vi "Scripting.vi"() -> ()   [LabVIEW 2019]
uses:
  NationalInstruments.VeriStand.SystemDefinitionAPI
  <vilib>/NI VeriStand/Custom Device API/Custom Device Item Ref.ctl
  Addon/Support Libraries/Protocols.lvlibp/Protocol Parent/Protocol Parent.lvclass
  Addon/Support Libraries/Protocols.lvlibp/TCP/TCP.lvclass
  Addon/Support Libraries/Protocols.lvlibp/UDP/UDP.lvclass
  Scripting API/Polymorphic/Create Message_TriggerOnly.vi
  Scripting API/Polymorphic/Create Message_PeriodicAndTrigger.vi
  Scripting API/Polymorphic/Create Message_ValueChangeAndTrigger.vi
  Scripting API/Polymorphic/Create Channel/Create Global Command Single Channel_Format.vi
  Scripting API/Polymorphic/Create Channel/Create Command Array Channel_Type Cast.vi
  Scripting API/Polymorphic/Add Response_Byte count.vi
  Scripting API/Polymorphic/Add Response_Wait sec.vi
  Scripting API/Polymorphic/Create Channel/Create Response Single Channel_Comparison.vi
  Scripting API/Scripting API.lvlib
  <vilib>/NI VeriStand/Custom Device API/Custom Device API.lvlib
  Scripting API/Polymorphic/Create RS-xxx.vi
  Scripting API/Polymorphic/Create TCP.vi
panel:
  out "Message refnum out 6":T1=18446744073709551615 format="%.0x"
  out "Channel refnum out 2":T1=18446744073709551615 format="%.0x"
  out "error out 17":errorcluster
  in  "Message refnum in 3":T1=18446744073709551615 format="%.0x"
  in  "Expected String":string
  in  "error in (no error) 17":errorcluster
  in  "Default Value 2":dbl
  in  "Units 2":string
  out "UDP out":refnum<class "UDP.lvclass">
  out "error out 13":errorcluster
  in  "error in (no error) 13":errorcluster
  out "TCP out":refnum<class "TCP.lvclass">
  out "error out 10":errorcluster
  in  "error in (no error) 10":errorcluster
  out "Response refnum out 2":T1=18446744073709551615 format="%.0x"
  out "error out 9":errorcluster
  in  "Response refnum in 2":T1=18446744073709551615 format="%.0x"
  in  "Response 2":string
  in  "Linkages 2":T2(array[cluster]) {"Linked Channel refnum" format="%.0x"}
  in  "error in (no error) 9":errorcluster
  in  "Wait value":dbl
  in  "Channel refnum 2":T1=18446744073709551615 format="%.0x"
  out "Response refnum out":T1=18446744073709551615 format="%.0x"
  out "error out 8":errorcluster
  in  "Response refnum in":T1=18446744073709551615 format="%.0x"
  in  "Response":string
  in  "Linkages":T2(array[cluster]) {"Linked Channel refnum" format="%.0x"}
  in  "error in (no error) 8":errorcluster
  in  "Byte Count value":u32
  in  "Channel refnum":T1=18446744073709551615 format="%.0x"
  out "Target out 4":refnum<k24>
  out "Instrument Addon Custom Device refnum 4":T1=18446744073709551615 format="%.0x"
  out "Message Channels refnums 4":T3 {"Enable Periodic" format="%.0x"; "Error Code" format="%.0x"; "Message Status" format="%.0x"; "Timestamp" format="%.0x"; "Trigger" format="%.0x"}
  out "error out 16":errorcluster
  in  "Target in 4":refnum<k24>
  in  "Protocol in":refnum<class "Protocol Parent.lvclass">
  in  "PCL Decimation 3":u16
  in  "error in (no error) 16":errorcluster
  out "Channel refnums out":T1[](array[typedef]) format="%.0x"
  out "Channel refnum out":T1=18446744073709551615 format="%.0x"
  out "Message refnum out 5":T1=18446744073709551615 format="%.0x"
  out "error out 15":errorcluster
  in  "Message refnum in 2":T1=18446744073709551615 format="%.0x"
  in  "Type":enum16{"DBL"}(ring)
  in  "Endian":enum16{"Big", "Little", "Native"}(ring)
  in  "error in (no error) 15":errorcluster
  in  "Delimiter":string
  out "Instrument Addon refnum out 3":T1=18446744073709551615 format="%.0x"
  out "error out 14":errorcluster
  in  "Instrument Addon refnum in 3":T1=18446744073709551615 format="%.0x"
  in  "Format String":string
  in  "error in (no error) 14":errorcluster
  in  "Default Value":dbl
  in  "Units":string
  in  "Trigger Channel refnum 3":T1=18446744073709551615 format="%.0x"
  in  "Enable Periodic Default ON 3":bool
  in  "Trigger Channel refnum 2":T1=18446744073709551615 format="%.0x"
  in  "Enable Periodic Default ON 2":bool
  in  "Trigger Channel refnum":T1=18446744073709551615 format="%.0x"
  in  "Enable Periodic Default ON":bool
  out "Message Channels refnums 3":T3 {"Enable Periodic" format="%.0x"; "Error Code" format="%.0x"; "Message Status" format="%.0x"; "Timestamp" format="%.0x"; "Trigger" format="%.0x"}
  out "Message Channels refnums 2":T3 {"Enable Periodic" format="%.0x"; "Error Code" format="%.0x"; "Message Status" format="%.0x"; "Timestamp" format="%.0x"; "Trigger" format="%.0x"}
  out "Message Channels refnums":T3 {"Enable Periodic" format="%.0x"; "Error Code" format="%.0x"; "Message Status" format="%.0x"; "Timestamp" format="%.0x"; "Trigger" format="%.0x"}
  out "Message Group refnum out 4":T1=18446744073709551615 format="%.0x"
  out "Message refnum out 4":T1=18446744073709551615 format="%.0x"
  out "error out 12":errorcluster
  in  "Message Group refnum in 3":T1=18446744073709551615 format="%.0x"
  in  "Message name 3":string
  in  "Protection 3":T4(ring)
  in  "error in (no error) 12":errorcluster
  out "Message Group refnum out 3":T1=18446744073709551615 format="%.0x"
  out "Message refnum out 3":T1=18446744073709551615 format="%.0x"
  out "error out 11":errorcluster
  in  "Message Group refnum in 2":T1=18446744073709551615 format="%.0x"
  in  "Message name 2":string
  in  "Protection 2":T4(ring)
  in  "error in (no error) 11":errorcluster
  in  "Period (sec)":u32
  out "Message Group refnum out 2":T1=18446744073709551615 format="%.0x"
  out "Message refnum out":T1=18446744073709551615 format="%.0x"
  out "error out 6":errorcluster
  in  "Message Group refnum in":T1=18446744073709551615 format="%.0x"
  in  "Message name":string
  in  "error in (no error) 6":errorcluster
  out "Command refnum out":T1=18446744073709551615 format="%.0x"
  out "Message refnum out 2":T1=18446744073709551615 format="%.0x"
  out "error out 7":errorcluster
  in  "Message refnum in":T1=18446744073709551615 format="%.0x"
  in  "Command":string
  in  "error in (no error) 7":errorcluster
  out "Instrument Addon refnum out 2":T1=18446744073709551615 format="%.0x"
  out "Message Group refnum out":T1=18446744073709551615 format="%.0x"
  out "error out 5":errorcluster
  in  "Instrument Addon refnum in 2":T1=18446744073709551615 format="%.0x"
  in  "Message Group name":string
  in  "error in (no error) 5":errorcluster
  out "Instrument Addon refnum out":T1=18446744073709551615 format="%.0x"
  out "error out 4":errorcluster
  in  "Instrument Addon refnum in":T1=18446744073709551615 format="%.0x"
  in  "Exported File path":path
  in  "error in (no error) 4":errorcluster
  out "Target out 3":refnum<k24>
  out "Instrument Addon Custom Device refnum 3":T1=18446744073709551615 format="%.0x"
  out "error out 3":errorcluster
  in  "Target in 3":refnum<k24>
  in  "Config File Path":path
  in  "error in (no error) 3":errorcluster
  out "Target out 2":refnum<k24>
  out "Instrument Addon Custom Device refnum 2":T1=18446744073709551615 format="%.0x"
  out "error out 2":errorcluster
  in  "Target in 2":refnum<k24>
  in  "PCL Decimation 2":u16
  in  "error in (no error) 2":errorcluster
  out "Target out":refnum<k24>
  out "Instrument Addon Custom Device refnum":T1=18446744073709551615 format="%.0x"
  out "error out":errorcluster
  in  "Target in":refnum<k24>
  in  "PCL Decimation":u16
  in  "error in (no error)":errorcluster
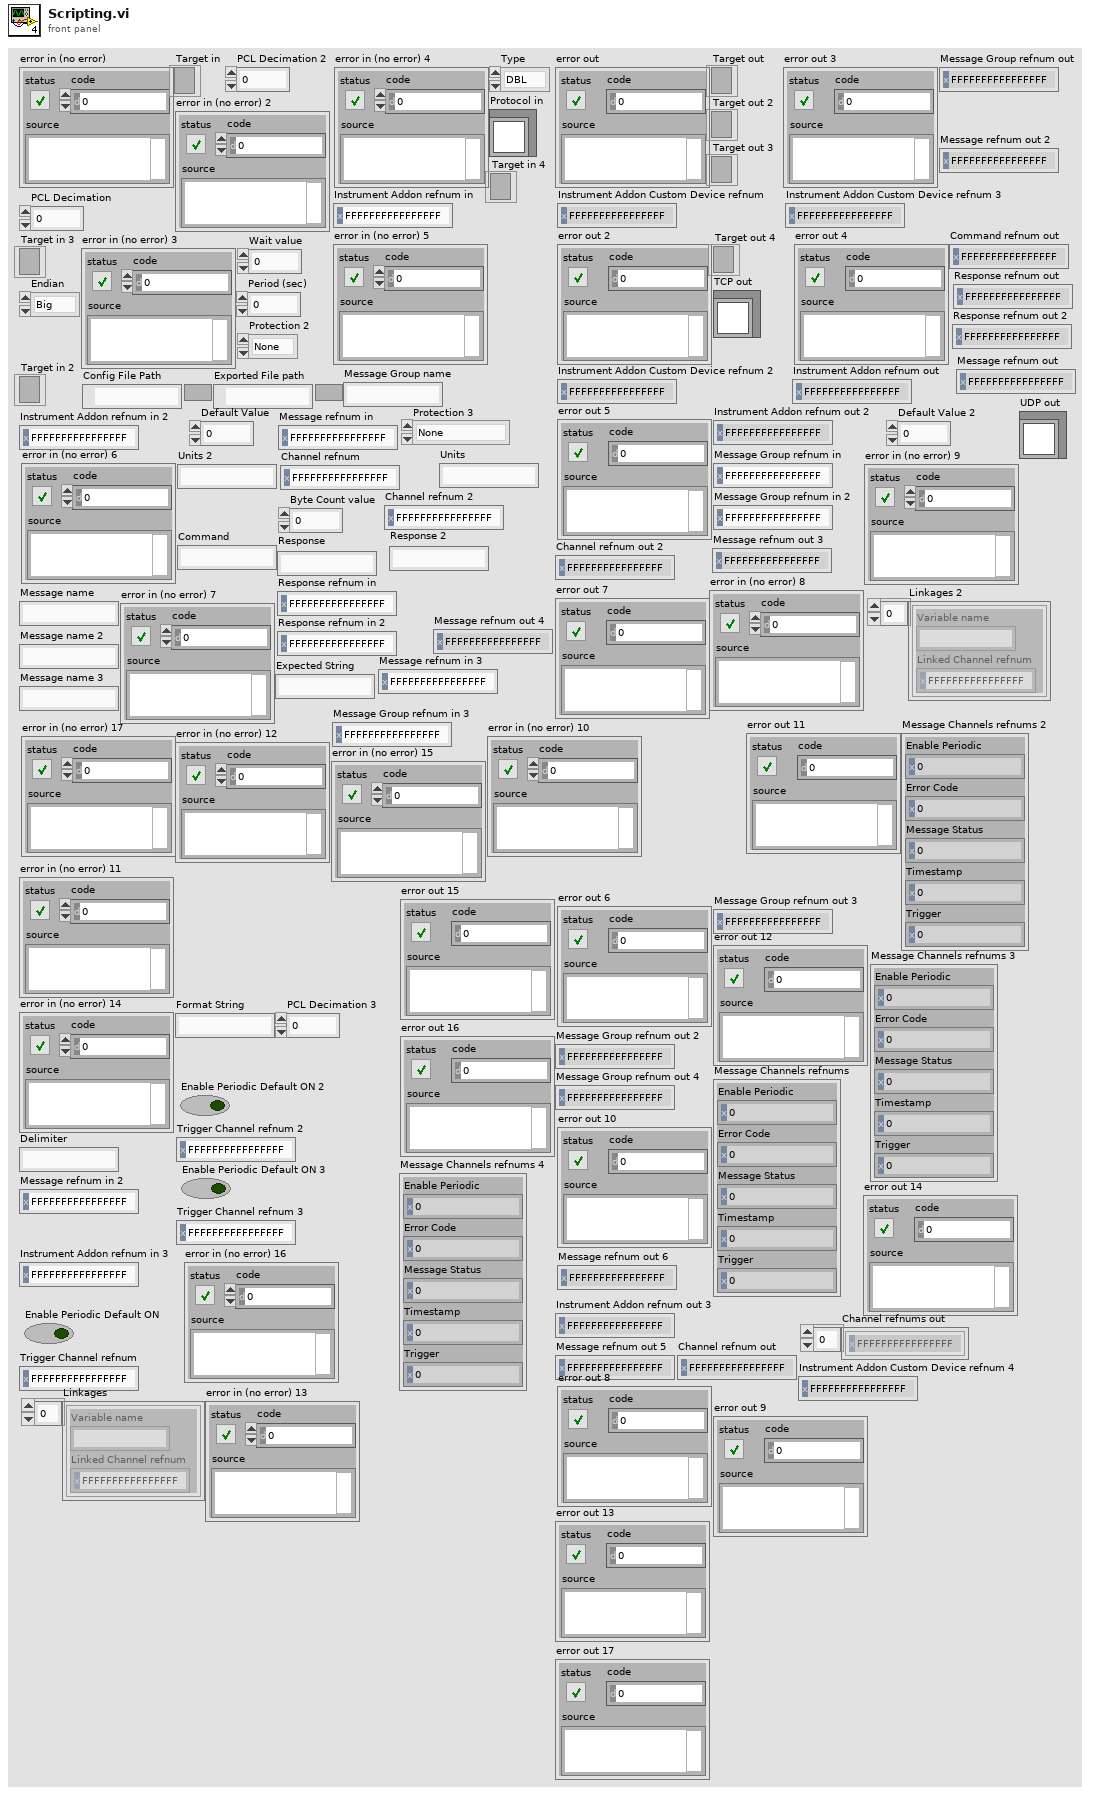
[diagram p1: front panel]
types:
  T1 = typedef "Custom Device API.lvlib/Custom Device Item Ref.ctl" = u64
  T2 = cluster{"Variable name":string, "Linked Channel refnum":T1}[]
  T3 = cluster{"Enable Periodic":T1, "Error Code":T1, "Message Status":T1, "Timestamp":T1, "Trigger":T1}
  T4 = enum16{"None", "CRC-32", "Checksum U8", "Checksum U16", "Checksum U32"}
  T5 = cluster{"Local IP Address":string, "Local Port":u16, "Target IP Address":string, "Target Port":u16}
  T6 = cluster{"Numeric":string, "Port":dbl, "Another Numeric":dbl, "Boolean":bool, "String":string}
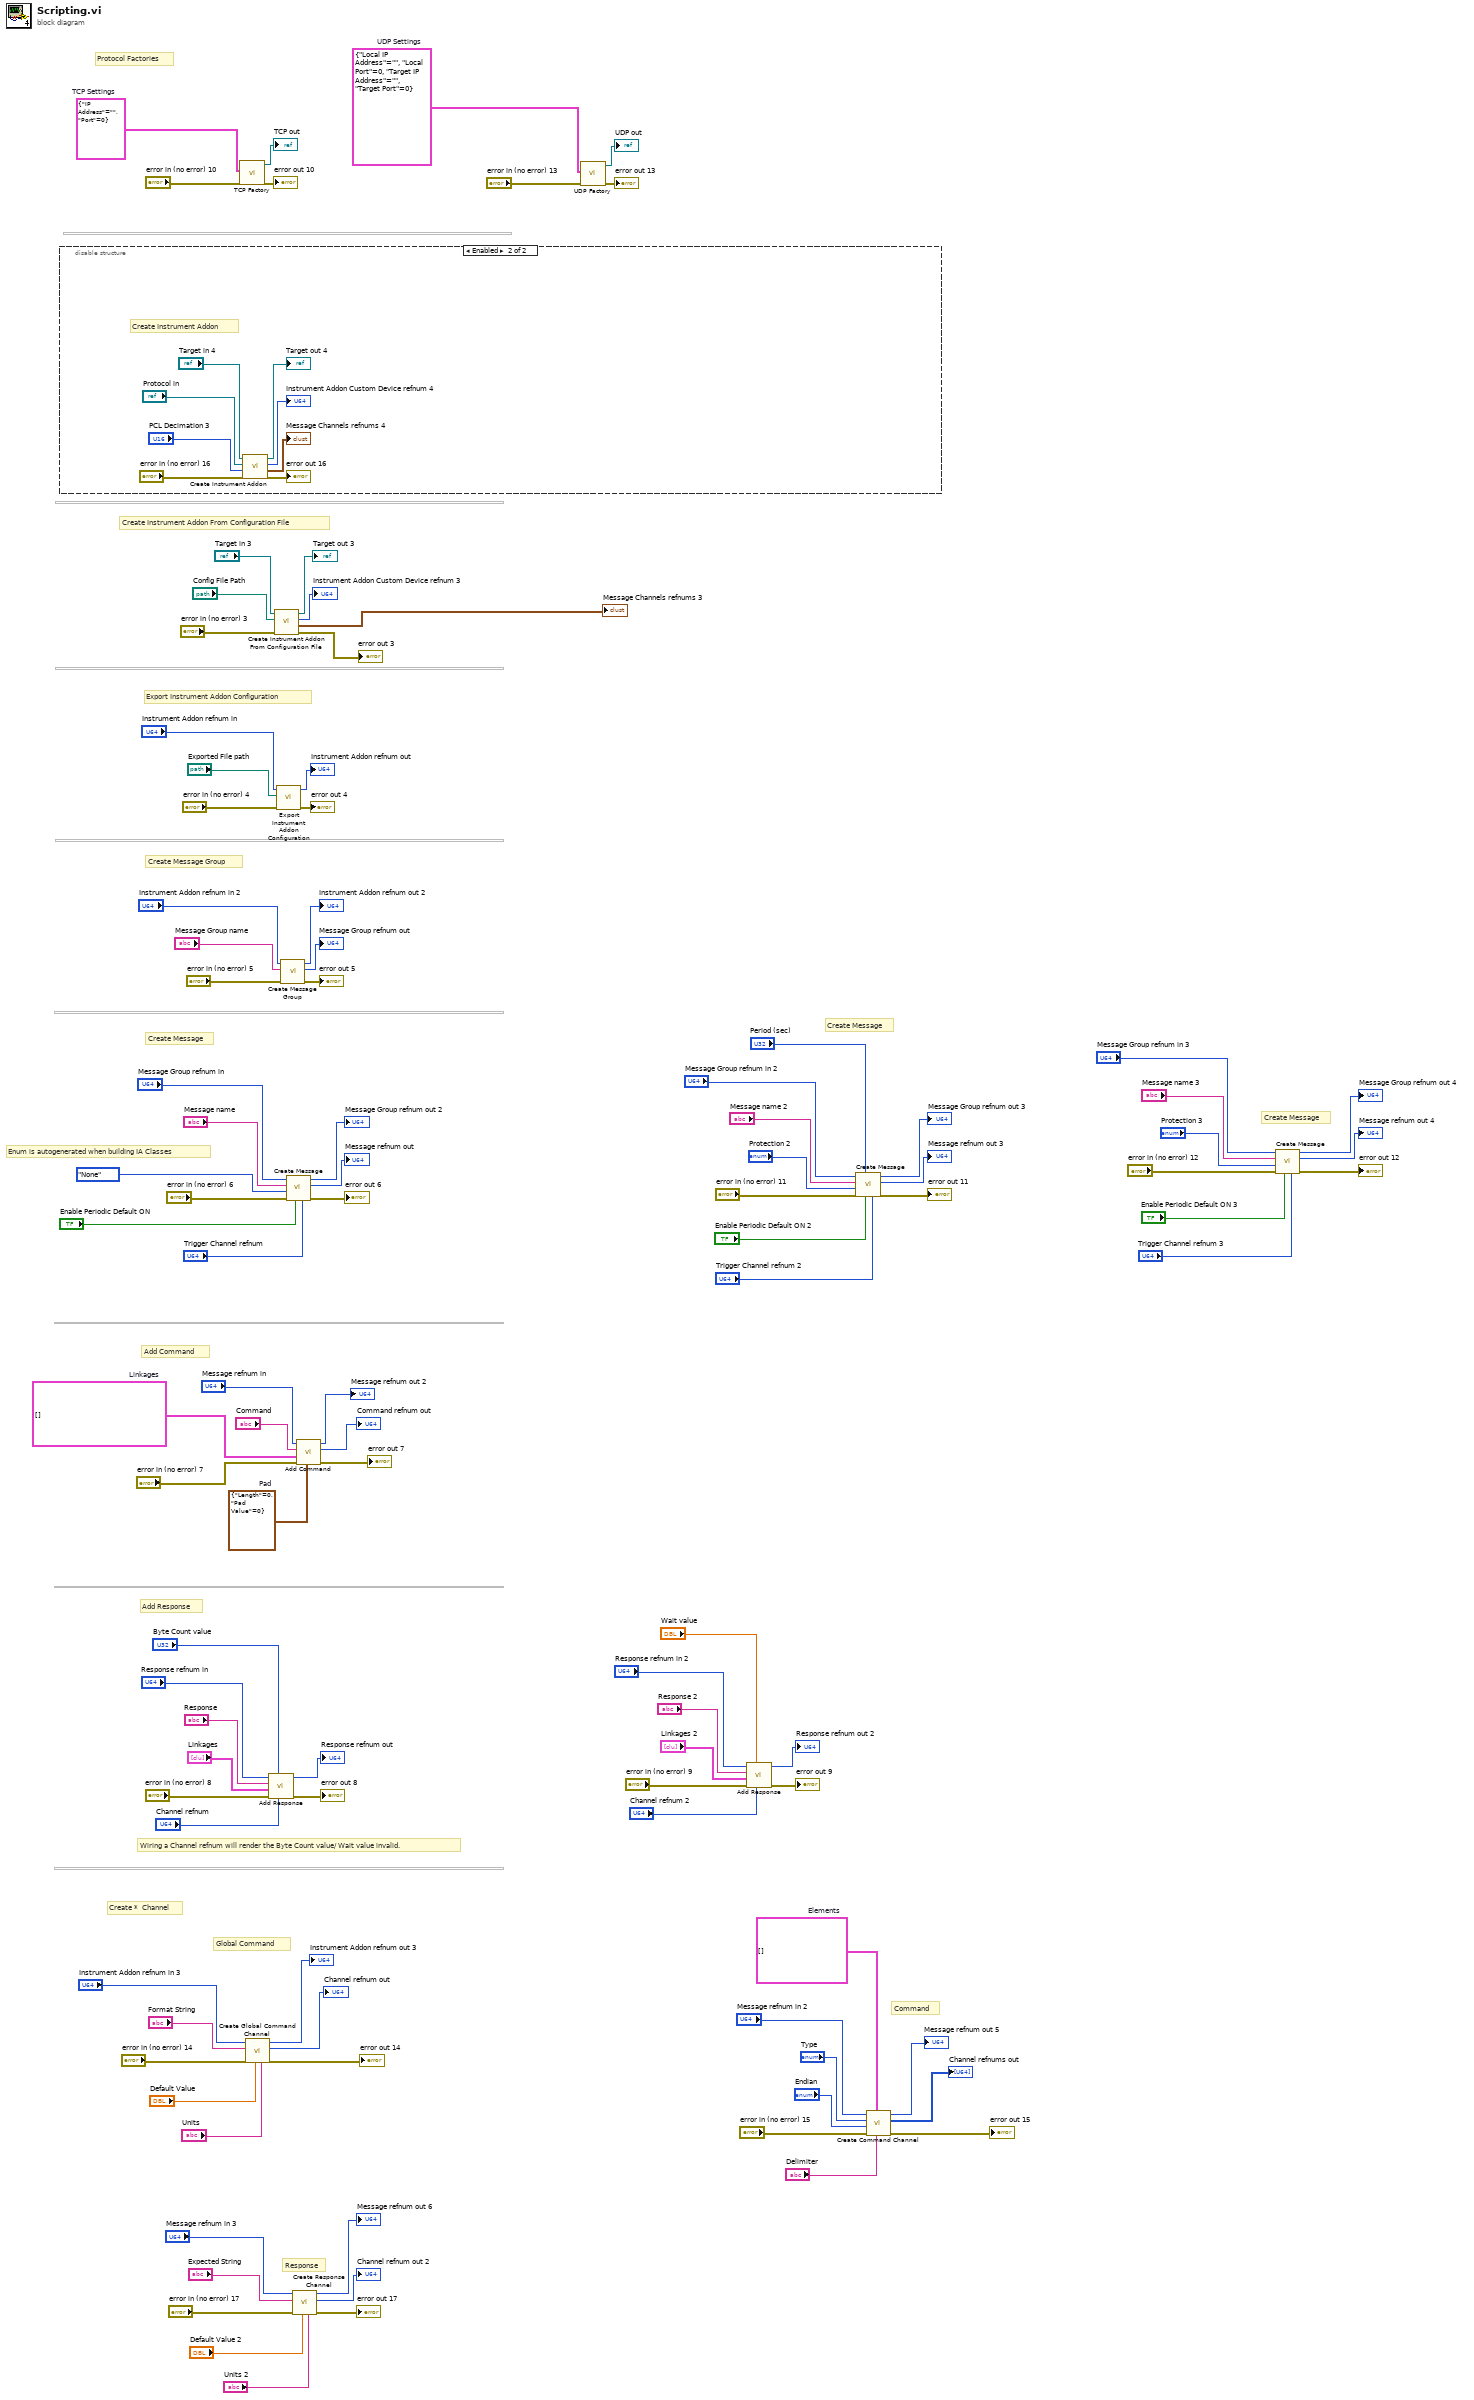
[diagram p0: block diagram]
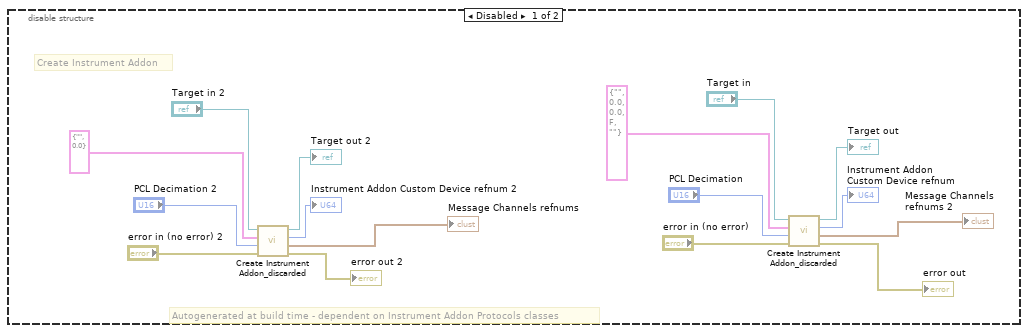
[diagram p2: hidden frame]
diagram:
  w11 = T5 {"Local IP Address"="", "Local Port"=0, "Target IP Address"="", "Target Port"=0}  # UDP Settings
  w15 = cluster{"IP Address":string, "Port":u16} {"IP Address"="", "Port"=0}  # TCP Settings
  w33 = T2 []  # Linkages
  w42 = cluster{"Default Value":dbl, "Units":string}[] []  # Elements
  w86 = cluster{"Length":u16, "Pad Value":u16} {"Length"=0, "Pad Value"=0}  # Pad
  # "Create Message"
  # "Create Message"
  # "Protocol Factories"
  # "Response"
  # "Command"
  # "Global Command"
  # "Create *  Channel"
  # "Enum is autogenerated when building IA Classes"
  # "Wiring a Channel refnum will render the Byte Count value/ Wait value invalid."
  # "Add Response"
  # "Add Command"
  # "Create Message"
  # "Create Message Group"
  # "Export Instrument Addon Configuration"
  # "Create Instrument Addon From Configuration File"
  n1 = disable-structure shown="Enabled" {
    frame Disabled {
      # "Autogenerated at build time - dependent on Instrument Addon Protocols classes"
      # "Create Instrument Addon"
      n2 = call-poly "Create Instrument Addon_discarded.vi"("error in (no error)"="error in (no error) 2", "PCL Decimation"="PCL Decimation 2", "Protocol Properties"=cluster{"IP Address":string, "Port":dbl} {"IP Address"="", "Port"=0.0}, "Target in"="Target in 2") -> ("error out"=→"error out 2":errorcluster, "Message Channels refnums"=→"Message Channels refnums":T3, "Instrument Addon Custom Device refnum"=→"Instrument Addon Custom Device refnum 2":T1, "Target out"=→"Target out 2":refnum<k24>)  [unwired: 4 in]
      n3 = call-poly "Create Instrument Addon_discarded.vi"("error in (no error)"="error in (no error)", "PCL Decimation"="PCL Decimation", "Protocol Properties"=T6 {"Numeric"="", "Port"=0.0, "Another Numeric"=0.0, "Boolean"=FALSE, "String"=""}, "Target in"="Target in") -> ("error out"=→"error out":errorcluster, "Message Channels refnums"=→"Message Channels refnums 2":T3, "Instrument Addon Custom Device refnum"=→"Instrument Addon Custom Device refnum":T1, "Target out"=→"Target out":refnum<k24>)  [unwired: 4 in]
    }
    frame Enabled {
      # "Create Instrument Addon"
      n4 = call "Create Instrument Addon.vi"("error in (no error)"="error in (no error) 16", "PCL Decimation"="PCL Decimation 3", "Protocol in"="Protocol in", "Target in"="Target in 4") -> ("error out"=→"error out 16":errorcluster, "Message Channels refnums"=→"Message Channels refnums 4":T3, "Instrument Addon Custom Device refnum"=→"Instrument Addon Custom Device refnum 4":T1, "Target out"=→"Target out 4":refnum<k24>)  [unwired: 4 in]
    }
  }
  n5 = call "TCP Factory.vi"("error in (no error)"="error in (no error) 10", "TCP Settings"=w15) -> ("error out"=→"error out 10":errorcluster, "TCP out"=→"TCP out":refnum<class "TCP.lvclass">)  [unwired: 8 in]
  n6 = call-poly "Create Global Command Channel.vi"("Units"="Units", "Default Value"="Default Value", "error in (no error)"="error in (no error) 14", "Format String"="Format String", "Instrument Addon refnum in"="Instrument Addon refnum in 3") -> ("error out"=→"error out 14":errorcluster, "Channel refnum out"=→"Channel refnum out":T1, "Instrument Addon refnum out"=→"Instrument Addon refnum out 3":T1)  [unwired: 4 in]
  n7 = call-poly "Add Response.vi"("Channel refnum"="Channel refnum", "Byte Count value"="Byte Count value", "error in (no error)"="error in (no error) 8", "Linkages"="Linkages", "Response"="Response", "Response refnum in"="Response refnum in") -> ("error out"=→"error out 8":errorcluster, "Response refnum out"=→"Response refnum out":T1)  [unwired: 4 in]
  n8 = call "Create Instrument Addon From Configuration File.vi"("error in (no error)"="error in (no error) 3", "Config File Path"="Config File Path", "Target in"="Target in 3") -> ("error out"=→"error out 3":errorcluster, "Message Channels refnums"=→"Message Channels refnums 3":T3, "Instrument Addon Custom Device refnum"=→"Instrument Addon Custom Device refnum 3":T1, "Target out"=→"Target out 3":refnum<k24>)  [unwired: 5 in]
  n9 = call "Export Instrument Addon Configuration.vi"("error in (no error)"="error in (no error) 4", "Exported File path"="Exported File path", "Instrument Addon refnum in"="Instrument Addon refnum in") -> ("error out"=→"error out 4":errorcluster, "Instrument Addon refnum out"=→"Instrument Addon refnum out":T1)  [unwired: 7 in]
  n10 = call "Create Message Group.vi"("error in (no error)"="error in (no error) 5", "Message Group name"="Message Group name", "Instrument Addon refnum in"="Instrument Addon refnum in 2") -> ("error out"=→"error out 5":errorcluster, "Message Group refnum out"=→"Message Group refnum out":T1, "Instrument Addon refnum out"=→"Instrument Addon refnum out 2":T1)  [unwired: 6 in]
  n11 = call-poly "Create Message.vi"("Trigger Channel refnum"="Trigger Channel refnum", "Enable Periodic Default ON"="Enable Periodic Default ON", "error in (no error)"="error in (no error) 6", "Protection"=T4."None", "Message name"="Message name", "Message Group refnum in"="Message Group refnum in") -> ("error out"=→"error out 6":errorcluster, "Message refnum out"=→"Message refnum out":T1, "Message Group refnum out"=→"Message Group refnum out 2":T1)  [unwired: 3 in]
  n12 = call-poly "Create Response Channel.vi"("Units"="Units 2", "Default Value"="Default Value 2", "error in (no error)"="error in (no error) 17", "Expected String"="Expected String", "Message refnum in"="Message refnum in 3") -> ("error out"=→"error out 17":errorcluster, "Channel refnum out"=→"Channel refnum out 2":T1, "Message refnum out"=→"Message refnum out 6":T1)  [unwired: 4 in]
  n13 = call "Add Command.vi"("Pad"=w86, "error in (no error)"="error in (no error) 7", "Linkages"=w33, "Command"="Command", "Message refnum in"="Message refnum in") -> ("error out"=→"error out 7":errorcluster, "Command refnum out"=→"Command refnum out":T1, "Message refnum out"=→"Message refnum out 2":T1)  [unwired: 4 in]
  n14 = call "UDP Factory.vi"("error in (no error)"="error in (no error) 13", "UDP Settings"=w11) -> ("error out"=→"error out 13":errorcluster, "UDP out"=→"UDP out":refnum<class "UDP.lvclass">)  [unwired: 8 in]
  n15 = call-poly "Add Response.vi"("Channel refnum"="Channel refnum 2", "Wait value"="Wait value", "error in (no error)"="error in (no error) 9", "Linkages"="Linkages 2", "Response"="Response 2", "Response refnum in"="Response refnum in 2") -> ("error out"=→"error out 9":errorcluster, "Response refnum out"=→"Response refnum out 2":T1)  [unwired: 4 in]
  n16 = call-poly "Create Message.vi"("Trigger Channel refnum"="Trigger Channel refnum 2", "Enable Periodic Default ON"="Enable Periodic Default ON 2", "Period (sec)"="Period (sec)", "error in (no error)"="error in (no error) 11", "Protection"="Protection 2", "Message name"="Message name 2", "Message Group refnum in"="Message Group refnum in 2") -> ("error out"=→"error out 11":errorcluster, "Message refnum out"=→"Message refnum out 3":T1, "Message Group refnum out"=→"Message Group refnum out 3":T1)  [unwired: 2 in]
  n17 = call-poly "Create Command Channel.vi"("Delimiter"="Delimiter", "Elements"=w42, "error in (no error)"="error in (no error) 15", "Endian"="Endian", "Type"="Type", "Message refnum in"="Message refnum in 2") -> ("error out"=→"error out 15":errorcluster, "Channel refnums out"=→"Channel refnums out":T1[], "Message refnum out"=→"Message refnum out 5":T1)  [unwired: 3 in]
  n18 = call-poly "Create Message.vi"("Trigger Channel refnum"="Trigger Channel refnum 3", "Enable Periodic Default ON"="Enable Periodic Default ON 3", "error in (no error)"="error in (no error) 12", "Protection"="Protection 3", "Message name"="Message name 3", "Message Group refnum in"="Message Group refnum in 3") -> ("error out"=→"error out 12":errorcluster, "Message refnum out"=→"Message refnum out 4":T1, "Message Group refnum out"=→"Message Group refnum out 4":T1)  [unwired: 3 in]
